vi "Event--Value Change.vi"(8 "error in":errorcluster, 11 "Selector in":refnum<class "Selector.lvclass">) -> (0 "error out":errorcluster, 2 "Name":string, 3 "Selector out":refnum<class "Selector.lvclass">)   [LabVIEW 2019, in "Selector.lvclass"]
uses:
  Selector.lvclass
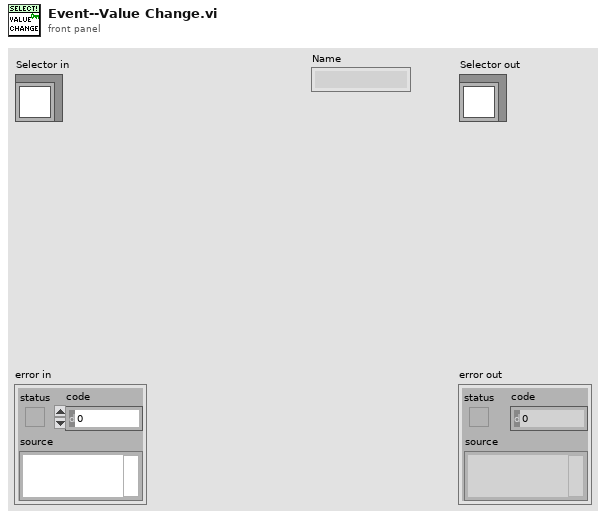
[diagram p1: front panel]
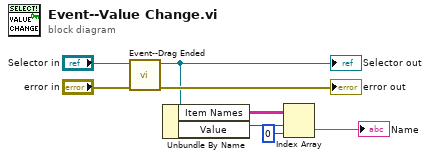
[diagram p0: block diagram]
diagram:
  n1 = call "Event--Drag Ended.vi"("error in"="error in", "Selector in"="Selector in") -> ("error out"=→"error out":errorcluster, "Selector out"=w5:refnum<class "Selector.lvclass">)  [unwired: 8 in]
  "Selector out" <- w5
  n2 = Unbundle By Name(w5) -> ("Item Names"=w4:string[][], "Value"=w3:i32)
  n3 = Index Array(array=w4, index (row)=w3, index (col)=0 ("disabled index (col)")) -> (element=→"Name":string)
